vi "FTDI SPI GPIO Read.vi"(4 "nCS":u8 max=4 step=1, 6 "ClockRate":u32=50000, 7 "Use Extra":bool, 9 "Addr":T1 items=["Addr-0", "Addr-1", "Addr-2", "Addr-3", "Addr-4", "Addr-5", "Addr-6"], 10 "Handler In":u32) -> (0 "error out":errorcluster, 1 "READ Reg B":u16, 2 "READ Reg A":u16, 3 "Handler Out":u32)   [LabVIEW 2018]
uses:
  PROJEKT/NIKO/Labview/Niko V4/FTDI SPI/Ctl/Sub Addr.ctl
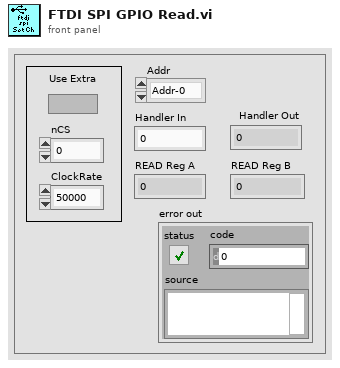
[diagram p1: front panel]
types:
  T1 = typedef "Sub Addr.ctl" = u16
  T2 = cluster{"ClockRate":u32, "LatencyTimer":u8, "configOptions 24-31":i8, "configOptions 16-23":i8, "configOptions 8-15":i8, "configOptions 0-7":u32, "Pin":u32, "reserved":u16}
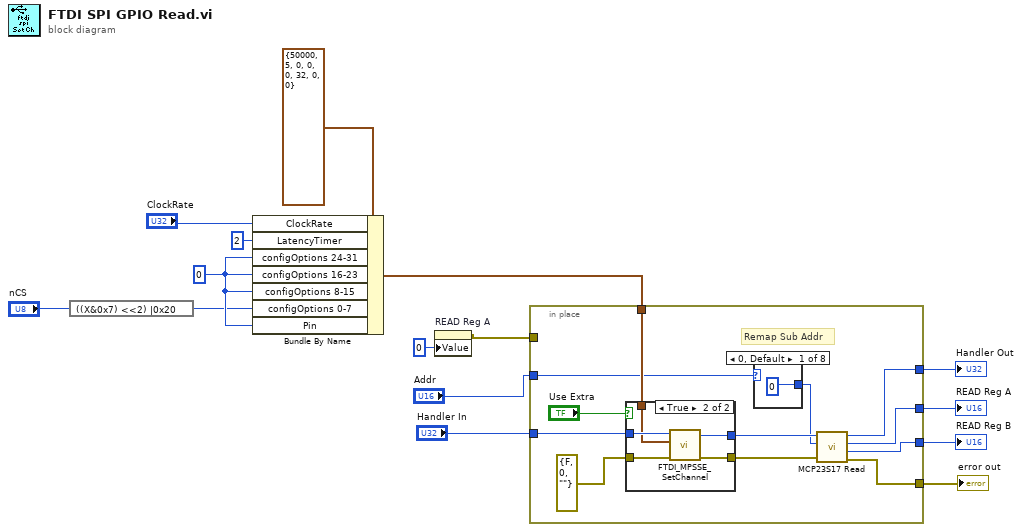
[diagram p0: block diagram]
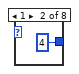
[diagram p2: hidden frame]
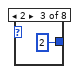
[diagram p3: hidden frame]
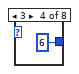
[diagram p4: hidden frame]
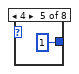
[diagram p5: hidden frame]
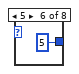
[diagram p6: hidden frame]
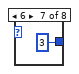
[diagram p7: hidden frame]
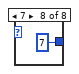
[diagram p8: hidden frame]
diagram:
  w7 = i8 0 ("configOptions 16-23")
  n1 = expression code="((X&0x7) <<2) |0x20"("nCS") -> (w5:u8)
  n2 = Bundle By Name(cluster=T2 {"ClockRate"=50000, "LatencyTimer"=5, "configOptions 24-31"=0, "configOptions 16-23"=0, "configOptions 8-15"=0, "configOptions 0-7"=32, "Pin"=0, "reserved"=0} ("config"), "ClockRate"="ClockRate", "LatencyTimer"=u8 2, "configOptions 24-31"=w7, "configOptions 16-23"=w7, "configOptions 8-15"=w7, "configOptions 0-7"=w5, "Pin"=w7) -> (w10:T2)
  n3 = property on="READ Reg A" class="DigNum (strict)"("Value"=u16 0 ("LATCH Reg")) -> (error out=w13:errorcluster)  [unwired: 2 in, 1 out]
  n4 = in-place {
    in-place-border: [w20] -> w15
    in-place-border: "Handler In" -> [w27]
    in-place-border: "Addr" -> [w23]
    in-place-border: w13 -> [_]
    in-place-border: w10 -> [w26]
    in-place-border: [w19] -> w3
    in-place-border: [w18] -> w2
    in-place-border: [w17] -> w1
    # "Remap Sub Addr"
    n5 = case shown="True" "Use Extra" {
      tunnel: w27 -> [w37 w42]
      tunnel: [w37 w41] -> w22
      tunnel: [w36 w40] -> w21
      tunnel: errorcluster {"status"=FALSE, "code"=0, "source"=""} ("error constant") -> [w36 w39]
      tunnel: w26 -> [_ w38]
      frame False {
      }
      frame True {
        n6 = call "FTDI_MPSSE_SetChannel.vi"("error in (no error)"=w39, "config"=w38, "handle"=w42) -> ("error out"=w40:errorcluster, "handle out"=w41:u32)  [unwired: 7 in]
      }
    }
    n7 = case shown="0, Default" w23 {
      tunnel: [0 4 2 6 1 5 3 7] -> w16
      frame 0, Default {
      }
      frame 1 {
      }
      frame 2 {
      }
      frame 3 {
      }
      frame 4 {
      }
      frame 5 {
      }
      frame 6 {
      }
      frame 7 {
      }
    }
    n8 = call "MCP23S17 Read.vi"("error in (no error)"=w21, "Addr"=w16, "handle"=w22) -> ("error out"=w20:errorcluster, "REG B"=w17:u16, "REG A"=w18:u16, "handle out"=w19:u32)  [unwired: 2 in, 2 out]
  }
  "Handler Out" <- w3
  "error out" <- w15
  "READ Reg A" <- w2
  "READ Reg B" <- w1
